vi "Receive.vi"(7 "Msg in":refnum<class "Msg Strategy.lvclass">, 11 "jettl State in":refnum<class "jettl State.lvclass">) -> (5 "Msg out":refnum<class "Msg Strategy.lvclass">)   [LabVIEW 2021, in "jettl.lvlib" / "jettl State.lvclass"]
uses:
  jettl State.lvclass
  Msg Strategy/Msg Strategy.lvclass
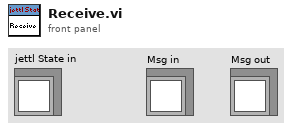
[diagram p1: front panel]
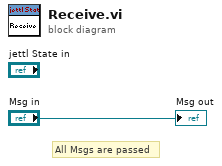
[diagram p0: block diagram]
diagram:
  # "All Msgs are passed"
  "Msg out" <- "Msg in"
